vi "Signal Breakout.vi"(0 "Pumps Enabled":bool[](array[boolean]), 5 "Tank Data":dbl[](array[numeric]), 7 "Intitial Times":dbl[](array[numeric])) -> (4 "Pump Data":T2={"Voltages"=[0.015201568603515625, 0.00335693359375, 0.003021240234375, 0.12260055541992188, 0.06085968017578125, 0.052234649658203125], "PumpCurrent"=[0.015201568603515625, 0.00335693359375, 0.003021240234375, 0.12260055541992188, 0.06085968017578125, 0.052234649658203125], "Speed"=[0.0, 0.0, 0.0, 0.0, 0.0, 0.0], "ControllerCurrent"=[0.015201568603515625, 0.00335693359375, 0.003021240234375, 0.12260055541992188, 0.06085968017578125, 0.052234649658203125], "Pressure"=[0.015201568603515625, 0.00335693359375, 0.003021240234375, 0.12260055541992188, 0.06085968017578125, 0.052234649658203125], "Flow"=[0.0, 0.0, 0.0, 0.125, 0.0625, 0.0625], "Elapsed Time:"=[7.1, 7.1, 7.1, 458133.45, 458138.85000000003, 458126.75], "Avg Pressure"=0.0} {"Elapsed Time:" format="%<%H:%M:%S>t"; "Speed" format="%#_4f"; "ControllerCurrent" format="%#.1g"; "Pressure" format="%#.0f"; "Flow" format="%#.0f"; "PumpCurrent" format="%#.1g"; "Voltages" format="%#.0f"}, 6 "Tank Data":T1 {"PS Actual (V):" format="%.2f"; "Temp1" format="%#_2g"; "Temp2" format="%#_2g"})   [LabVIEW 2013]
uses:
  Controls/Pump Data.ctl
  Controls/Tank Data.ctl
  Controls/Live Tank Data.ctl
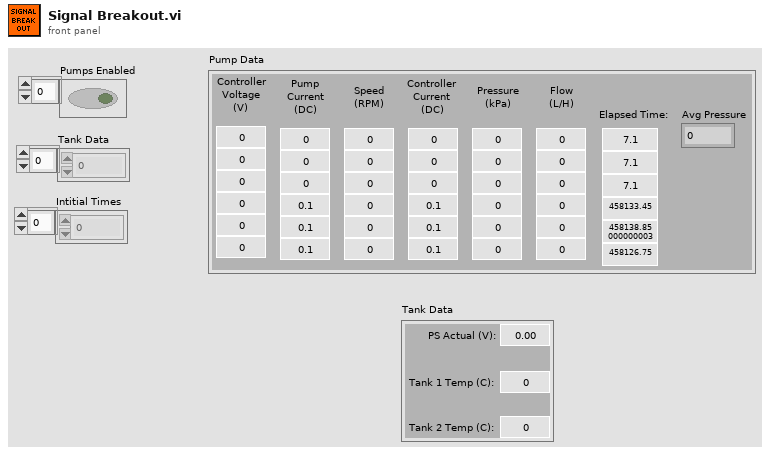
[diagram p1: front panel]
types:
  T1 = typedef "Tank Data.ctl" = cluster{"PS Actual (V):":dbl, "Temp1":dbl, "Temp2":dbl}
  T2 = typedef "Pump Data.ctl" = cluster{"Voltages":dbl[], "PumpCurrent":dbl[], "Speed":dbl[], "ControllerCurrent":dbl[], "Pressure":dbl[], "Flow":dbl[], "Elapsed Time:":dbl[], "Avg Pressure":dbl}
  T3 = typedef "Live Tank Data.ctl" = cluster{"PS Actual (V):":dbl, "Temp1":dbl, "Temp2":dbl}
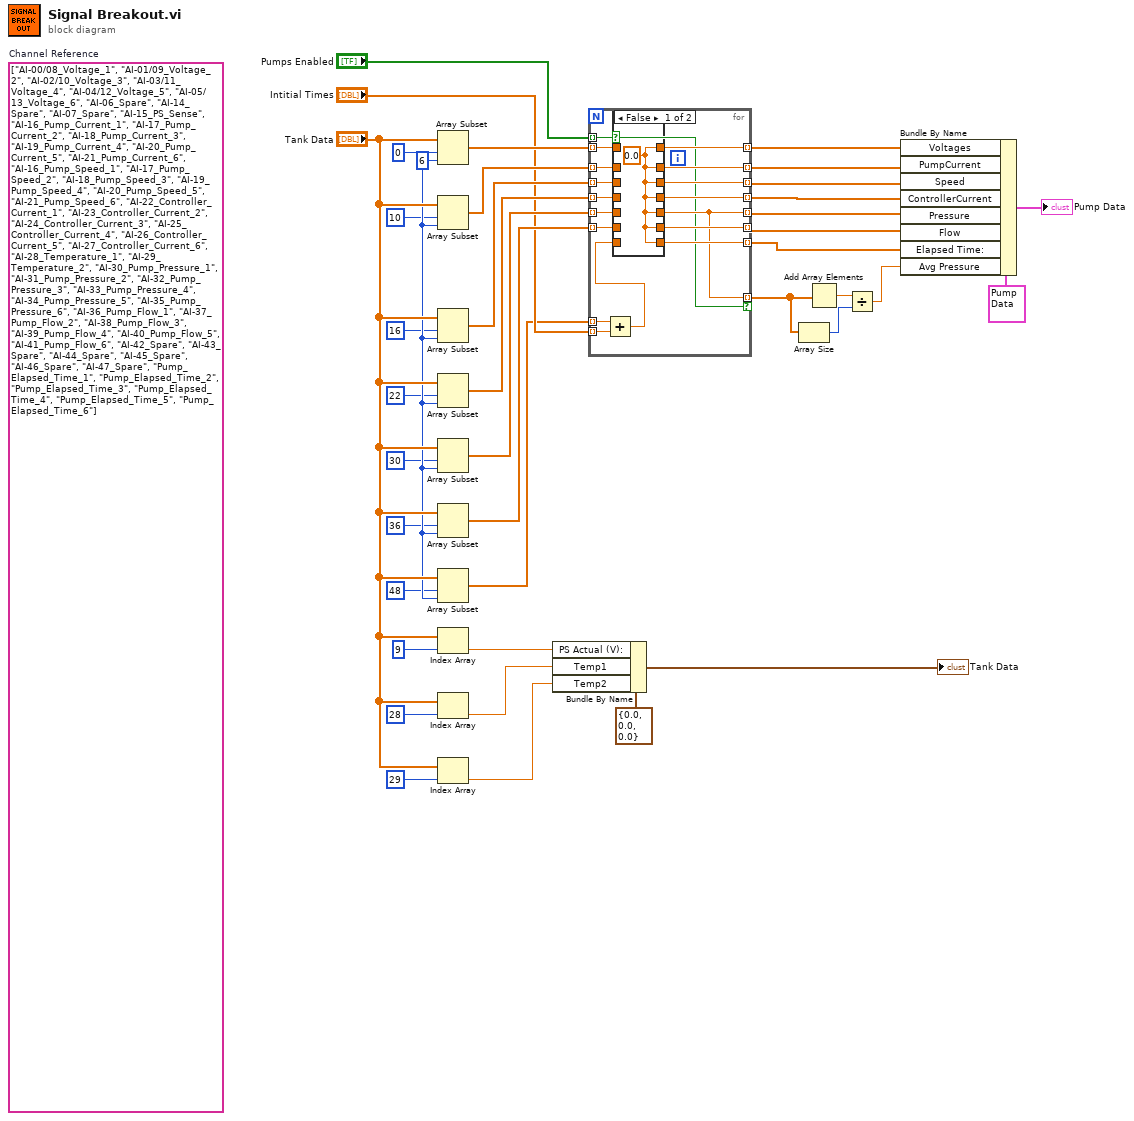
[diagram p0: block diagram]
diagram:
  w37 = 6 ("length")
  (unwired) string[] ["AI-00/08_Voltage_1", "AI-01/09_Voltage_2", "AI-02/10_Voltage_3", "AI-03/11_Voltage_4", "AI-04/12_Voltage_5", "AI-05/13_Voltage_6", "AI-06_Spare", "AI-14_Spare", "AI-07_Spare", "AI-15_PS_Sense", "AI-16_Pump_Current_1", "AI-17_Pump_Current_2", "AI-18_Pump_Current_3", "AI-19_Pump_Current_4", "AI-20_Pump_Current_5", "AI-21_Pump_Current_6", "AI-16_Pump_Speed_1", "AI-17_Pump_Speed_2", "AI-18_Pump_Speed_3", "AI-19_Pump_Speed_4", "AI-20_Pump_Speed_5", "AI-21_Pump_Speed_6", "AI-22_Controller_Current_1", "AI-23_Controller_Current_2", "AI-24_Controller_Current_3", "AI-25_Controller_Current_4", "AI-26_Controller_Current_5", "AI-27_Controller_Current_6", "AI-28_Temperature_1", "AI-29_Temperature_2", "AI-30_Pump_Pressure_1", "AI-31_Pump_Pressure_2", "AI-32_Pump_Pressure_3", "AI-33_Pump_Pressure_4", "AI-34_Pump_Pressure_5", "AI-35_Pump_Pressure_6", "AI-36_Pump_Flow_1", "AI-37_Pump_Flow_2", "AI-38_Pump_Flow_3", "AI-39_Pump_Flow_4", "AI-40_Pump_Flow_5", "AI-41_Pump_Flow_6", "AI-42_Spare", "AI-43_Spare", "AI-44_Spare", "AI-45_Spare", "AI-46_Spare", "AI-47_Spare", "Pump_Elapsed_Time_1", "Pump_Elapsed_Time_2", "Pump_Elapsed_Time_3", "Pump_Elapsed_Time_4", "Pump_Elapsed_Time_5", "Pump_Elapsed_Time_6"]  # Channel Reference
  n1 = Array Subset(array="Tank Data", index=0, length=w37) -> (w27:dbl[])
  n2 = Array Subset(array="Tank Data", index=10, length=w37) -> (w26:dbl[])
  n3 = Array Subset(array="Tank Data", index=16, length=w37) -> (w25:dbl[])
  n4 = Array Subset(array="Tank Data", index=22, length=w37) -> (w24:dbl[])
  n5 = Array Subset(array="Tank Data", index=30, length=w37) -> (w23:dbl[])
  n6 = Array Subset(array="Tank Data", index=36, length=w37) -> (w22:dbl[])
  n7 = Array Subset(array="Tank Data", index=48, length=w37) -> (w11:dbl[])
  n8 = Index Array(array="Tank Data", index=9) -> (element=w9:dbl)
  n9 = Index Array(array="Tank Data", index=28) -> (element=w8:dbl)
  n10 = Index Array(array="Tank Data", index=29) -> (element=w7:dbl)
  n11 = Bundle By Name(cluster=T3 {"PS Actual (V):"=0.0, "Temp1"=0.0, "Temp2"=0.0} ("Tank Data"), "PS Actual (V):"=w9, "Temp1"=w8, "Temp2"=w7) -> (→"Tank Data":T3)
  n12 = for {
    tunnel: w27 -> [w56] mode=indexing
    tunnel: [w55] -> w18 mode=indexing
    tunnel: w26 -> [w54] mode=indexing
    tunnel: w25 -> [w53] mode=indexing
    tunnel: w24 -> [w52] mode=indexing
    tunnel: w23 -> [w51] mode=indexing
    tunnel: w22 -> [w50] mode=indexing
    tunnel: w11 -> [w45] mode=indexing
    tunnel: [w49] -> w17 mode=indexing
    tunnel: [w48] -> w16 mode=indexing
    tunnel: [w47] -> w15 mode=indexing
    tunnel: [w41] -> w14 mode=indexing
    tunnel: [w46] -> w13 mode=indexing
    tunnel: "Pumps Enabled" -> [w40] mode=indexing
    tunnel: "Intitial Times" -> [w44] mode=indexing
    tunnel: [w42] -> w12 mode=indexing
    tunnel: [w41] -> w4 mode=indexing if=w40
    n13 = Add(x=w45, y=w44) -> (x+y=w43:dbl)
    n14 = case shown="False" w40 {
      tunnel: w56 -> [_ w64]
      tunnel: [w57 w64] -> w55
      tunnel: w54 -> [_ w63]
      tunnel: w53 -> [_ w62]
      tunnel: w52 -> [_ w61]
      tunnel: w51 -> [_ w60]
      tunnel: w50 -> [_ w59]
      tunnel: [w57 w63] -> w49
      tunnel: [w57 w62] -> w48
      tunnel: [w57 w61] -> w47
      tunnel: [w57 w60] -> w41
      tunnel: [w57 w59] -> w46
      tunnel: [w57 w58] -> w42
      tunnel: w43 -> [_ w58]
      frame False {
        w57 = 0.0
      }
      frame True {
      }
    }
  }
  n15 = Array Size(array=w4) -> (size(s)=w2:i32)
  n16 = Add Array Elements(numeric array=w4) -> (sum=w3:dbl)
  n17 = Divide(x=w3, y=w2) -> (x/y=w1:dbl)
  n18 = Bundle By Name(cluster=T2 {"Voltages"=[0.0, 0.05908203125, 0.06982421875, 0.05908203125, 0.06982421875, 0.0859375], "PumpCurrent"=[0.0015967955457961394, 0.0015950073791676203, 0.0015981739242389562, 0.0015920643549248493, 0.001590499709124895, 0.0015808510600251774], "Speed"=[0.0, 0.0, 0.0, 0.0, 0.0, 0.0], "ControllerCurrent"=[-20.688123176070036, -20.81007435196841, -20.6654170362211, -20.809705989642936, -20.754042150663764, -20.945938358319978], "Pressure"=[172.64492233694307, 172.85003218327398, 196.83234134789615, 194.272392502873, 196.0868331665868, 197.0256255267641], "Flow"=[114.82946701905468, 115.15906524483574, 115.40397142867363, 115.72441088850422, 113.53169391236554, 111.97984467984668], "Elapsed Time:"=[4074.9003000000002, 4074.9003000000002, 4074.9003000000002, 4074.9003000000002, 4074.9003000000002, 4074.9003000000002], "Avg Pressure"=0.0} ("Pump Data"), "Voltages"=w18, "PumpCurrent"=w17, "Speed"=w16, "ControllerCurrent"=w15, "Pressure"=w14, "Flow"=w13, "Elapsed Time:"=w12, "Avg Pressure"=w1) -> (→"Pump Data":T2)
